vi "ABC End.vi"(6 "UART":refnum<vi>, 7 "DaqTask":refnum<k21>, 8 "ErrIn":errorcluster, 11 "ComPort":refnum<visa-resource-name>) -> (0 "ErrOut":errorcluster)   [LabVIEW 2020]
uses:
  <userlib>/Amira UART/Amira UART.lvclass
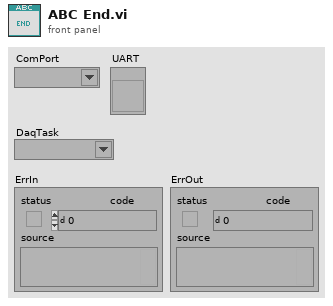
[diagram p1: front panel]
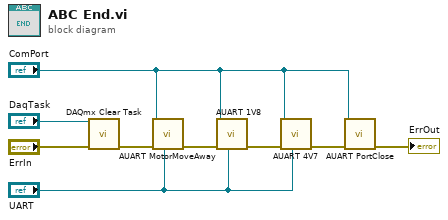
[diagram p0: block diagram]
diagram:
  n1 = call <vilib>:"DAQmx Clear Task.vi"("task in"="DaqTask", "error in"="ErrIn") -> ("error out"=w9:errorcluster)  [unwired: 13 in]
  n2 = call <userlib>:"AUART MotorMoveAway.vi"("UART"="UART", "ErrIn"=w9, "Port"="ComPort") -> ("ErrOut"=w5:errorcluster)  [unwired: 8 in]
  n3 = call <userlib>:"AUART 1V8.vi"("UART"="UART", "ErrIn"=w5, "Port"="ComPort") -> ("ErrOut"=w4:errorcluster)  [unwired: 7 in, 1 out]
  n4 = call <userlib>:"AUART 4V7.vi"("UART"="UART", "ErrIn"=w4, "Port"="ComPort") -> ("ErrOut"=w3:errorcluster)  [unwired: 7 in, 1 out]
  n5 = call <userlib>:"AUART PortClose.vi"("ErrIn"=w3, "Port"="ComPort") -> ("ErrOut"=→"ErrOut":errorcluster)  [unwired: 9 in]
